vi "Create New Build.vi"(7 "TargetItem Refnum":refnum<vi>, 8 "error in (no error)":errorcluster, 9 "Build specification name":string, 10 "Build object selector":T1, 11 "Project Refnum":refnum<vi>) -> (0 "error out":errorcluster, 3 "NI_AB_API_Build out":refnum<class "NI_AB_API_Build.lvclass">)   [LabVIEW 2020, in "NI_AB_API_Build.lvclass"]
uses:
  <vilib>/AppBuilder/AB_API/Build/NI_AB_API_Build.lvclass
  <vilib>/AppBuilder/AB_API/Build/NI_AB_API_Build.lvclass/NI_AB_API_Build.ctl
  <vilib>/AppBuilder/AB_Classes/Build/AB_Build.lvclass
  <vilib>/AppBuilder/AB_API/common/AB_API Build Object Selector.ctl
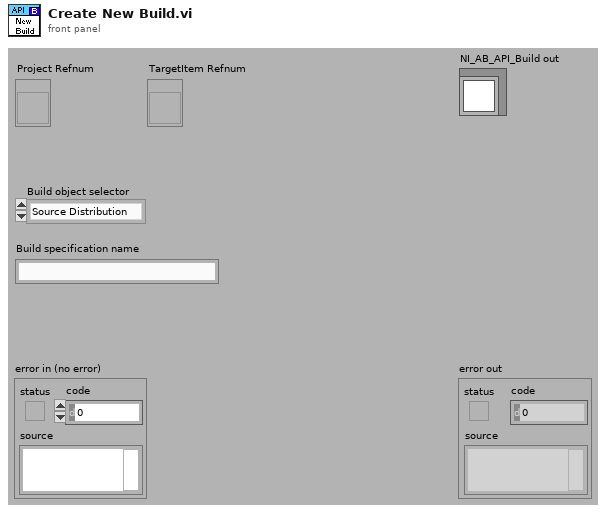
[diagram p1: front panel]
types:
  T1 = typedef "AB_API Build Object Selector.ctl" = enum16{"Source Distribution", "Deployable Source Distribution", "DLL", "EXE", "Packed Library", "Deployable Packed Library", "RT EXE", ".NET Interop Assembly"}
  T2 = typedef "AB_API Build Object Type.ctl" = enum16{"Source Distribution", "DLL", "EXE", "Installer", "Zip File", "RESTful WS", "RTEXE", "Packed Library", "C Generation ", ".NET Interop Assembly"}
  T3 = typedef "ItemRef.ctl" = u64
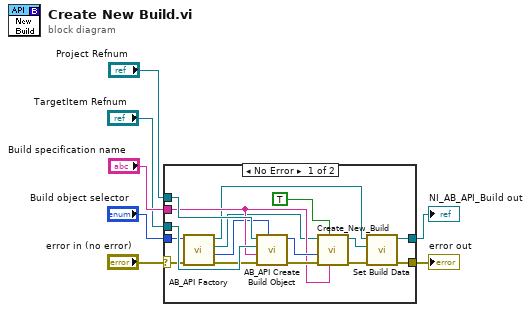
[diagram p0: block diagram]
diagram:
  n1 = case shown="No Error" "error in (no error)" {
    selector: "error in (no error)" -> [w9 w24]
    tunnel: [w16 w24] -> w6
    tunnel: [w14 _] -> w5
    tunnel: "Project Refnum" -> [w22 _]
    tunnel: "Build specification name" -> [w18 _]
    tunnel: "TargetItem Refnum" -> [w21 _]
    tunnel: "Build object selector" -> [w13 _]
    frame No Error {
      n2 = call <vilib>:"AB_API Factory.vi"("error in (no error)"=w9, "Build object selector"=w13) -> ("error out"=w8:errorcluster, "Build object type"=w10:T2, "Build"=w11:refnum<class "AB_Build.lvclass">, "API"=w12:refnum<class "NI_AB_API_Build.lvclass">)  [unwired: 6 in]
      n3 = call <vilib>:"AB_API Create Build Object.vi"("Build object type"=w10, "error in (no error)"=w8, "Build spec name"=w18, "TargetItem Refnum"=w21, "Project Refnum"=w22) -> ("error out"=w20:errorcluster, "Build object"=w19:T3)  [unwired: 5 out]
      n4 = call-dynamic "Create_New_Build.vi"("buildSpecName"=w18, "Programmatic? (false)"=TRUE, "error in (no error)"=w20, "buildObject"=w19, "AB_Build in"=w11) -> ("error out"=w17:errorcluster, "AB_Build out"=w15:refnum<class "AB_Build.lvclass">)  [unwired: 1 in, 4 out]
      n5 = call <vilib>:"Set Build Data.vi"("error in (no error)"=w17, "AB_Build.lvclass"=w15, "NI_AB_API_Build in"=w12) -> ("error out"=w16:errorcluster, "NI_AB_API_Build out"=w14:refnum<class "NI_AB_API_Build.lvclass">)  [unwired: 7 in]
    }
    frame Error {
    }
  }
  "error out" <- w6
  "NI_AB_API_Build out" <- w5
